vi "Write Key Boolean.vi"(6 "Insert If Not Exist(T)":bool=TRUE, 7 "Section Name":string, 8 "error in (no error)":errorcluster, 9 "Key Value":bool, 10 "Key Name":string, 11 "Config Data":T1(array[cluster])) -> (0 "error out":errorcluster, 3 "Config Data dup":T1(array[cluster]))   [LabVIEW 2020, in "GUCalibration2.lvlib"]
uses:
  GUCalibration2.lvlib
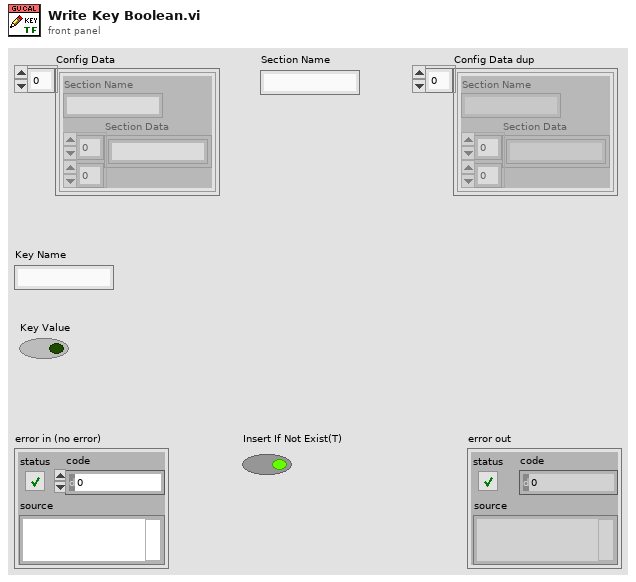
[diagram p1: front panel]
types:
  T1 = cluster{"Section Name":string, "Section Data":string[][]}[]
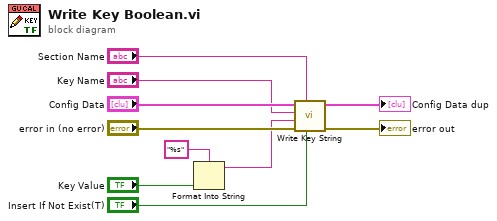
[diagram p0: block diagram]
diagram:
  n1 = Format Into String(format string="%s", "Key Value") -> (resulting string=w1:string)  [unwired: 2 in, 1 out]
  n2 = call "Write Key String.vi"("Insert If Not Exist(T)"="Insert If Not Exist(T)", "Section Name"="Section Name", "error in (no error)"="error in (no error)", "Key Value"=w1, "Key Name"="Key Name", "Config Data"="Config Data") -> ("error out"=→"error out":errorcluster, "Config Data dup"=→"Config Data dup":T1)  [unwired: 4 in]
